vi "to SGL.vi"(8 "error in":errorcluster, 11 "bytes":u8[](array[numeric]) format="%b") -> (0 "error out":errorcluster, 3 "SGL":sgl)   [LabVIEW 2020, in "wamplv.lvlib" / "MessagePack.lvclass"]
uses:
  MessagePack.lvclass
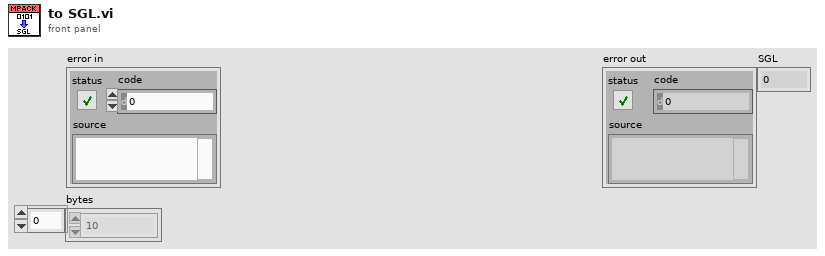
[diagram p1: front panel]
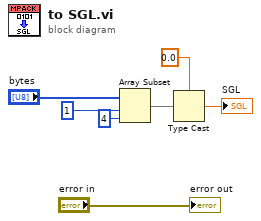
[diagram p0: block diagram]
diagram:
  n1 = Array Subset(array="bytes", index=1, length=4) -> (w1:u8[])
  n2 = Type Cast(type=sgl 0.0 ("SGL"), x=w1) -> (*(type *) &x=→"SGL":sgl)
  "error out" <- "error in"
